vi "RemoveScanFunc.vi"(0 "LoadedInstIn":refnum<class "BaseDevice.lvclass">[](array[class]), 1 "LoadedFuncArr":string[](array[string]), 2 "ScanFunc":string, 3 "Multi ScanPar":bool[](array[boolean]), 5 "ScanSubPan":refnum<vi>, 7 "WholeTask(No:T)":bool, 9 "ScanFuncArrIn":string[][](array[string]), 11 "ErrorIn(No Error)":errorcluster caption="entrée d'erreur (pas d'erreur)", 12 "ActScanPar":bool[](array[boolean]), 13 "TaskIdx":i32) -> (4 "LoadedInst":refnum<class "BaseDevice.lvclass">[](array[class]), 6 "Multi ScanParOut":bool[](array[boolean]), 10 "ScanFuncArrOut":string[][](array[string]), 14 "ActScanParOut":bool[](array[boolean]), 15 "sortie d'erreur":errorcluster)   [LabVIEW 2019]
uses:
  DevicesClass/BaseDevice/BaseDevice.lvclass
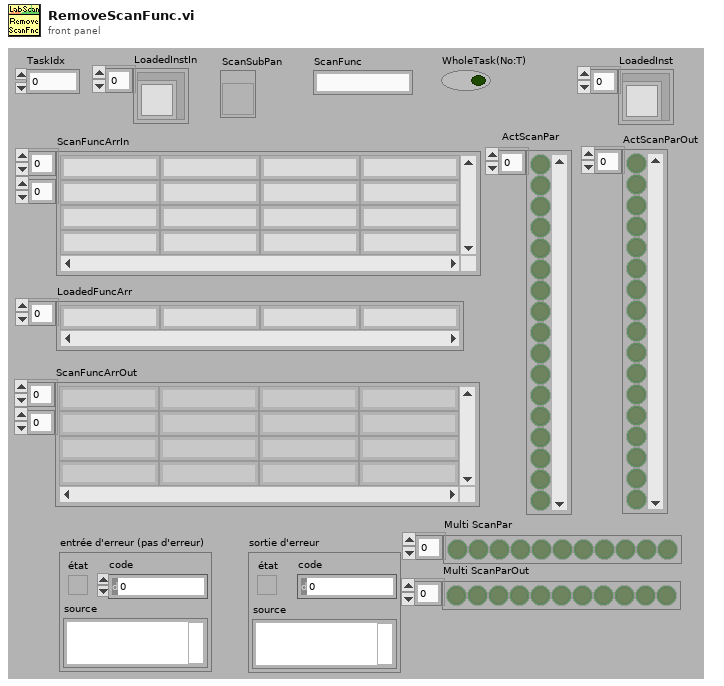
[diagram p1: front panel]
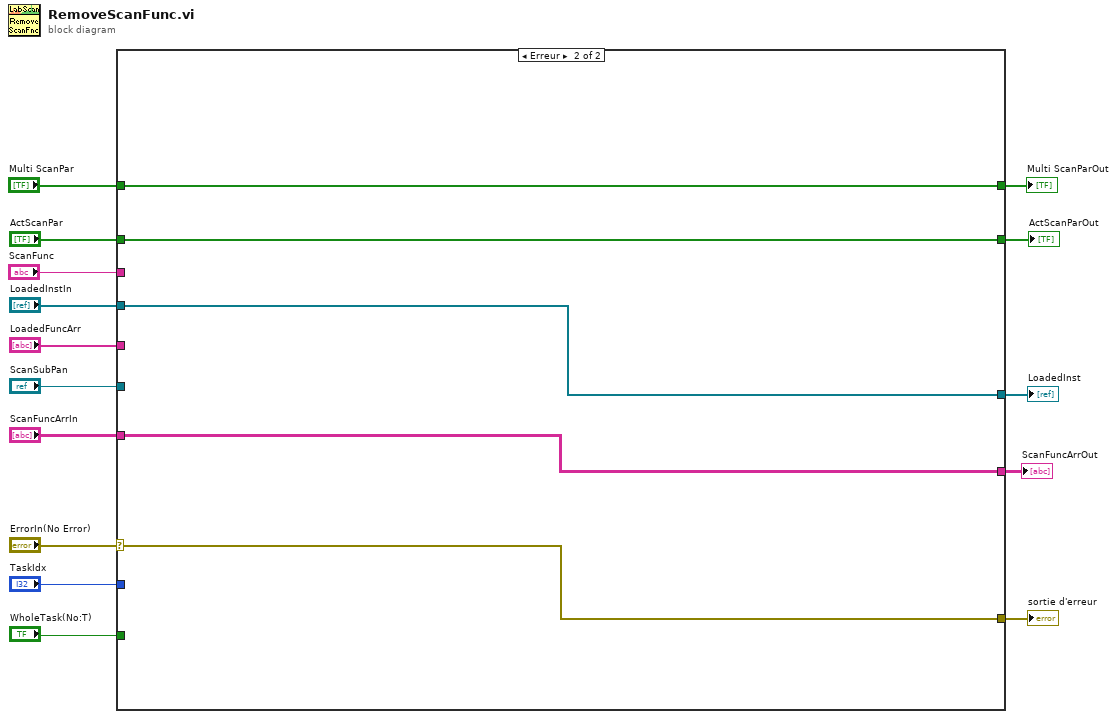
[diagram p0: block diagram]
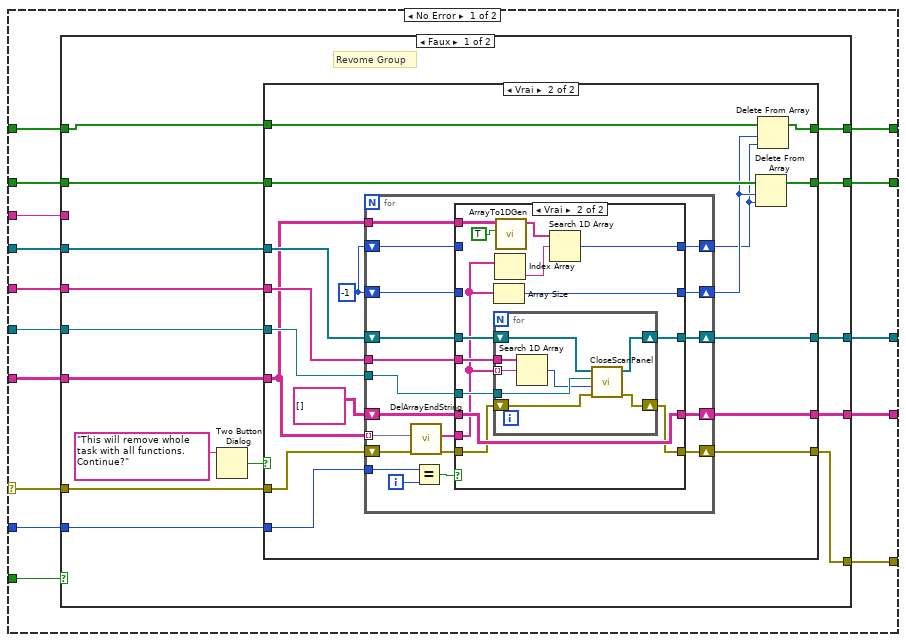
[diagram p2: hidden frame]
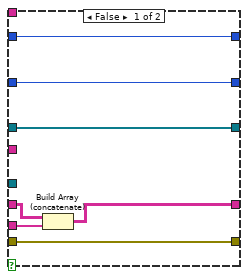
[diagram p4: hidden frame]
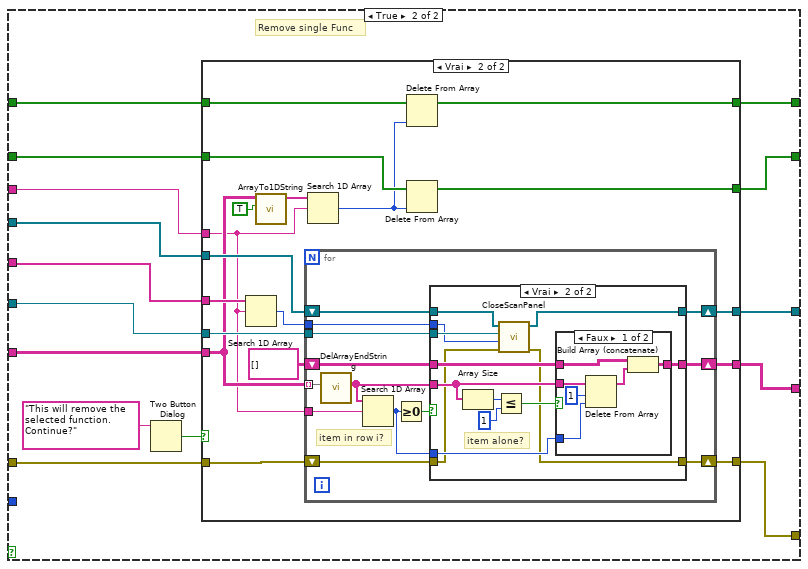
[diagram p5: hidden frame]
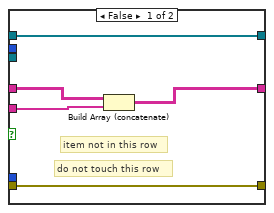
[diagram p7: hidden frame]
diagram:
  n1 = case shown="Erreur" "ErrorIn(No Error)" {
    selector: "ErrorIn(No Error)" -> [w30 w196]
    tunnel: "ScanFuncArrIn" -> [w27 w195]
    tunnel: "WholeTask(No:T)" -> [w28 _]
    tunnel: [w24 w196] -> w12
    tunnel: [w25 w195] -> w11
    tunnel: "ActScanPar" -> [w21 w194]
    tunnel: [w18 w194] -> w9
    tunnel: "TaskIdx" -> [w29 _]
    tunnel: [w26 w193] -> w7
    tunnel: "LoadedInstIn" -> [w23 w193]
    tunnel: "LoadedFuncArr" -> [w22 _]
    tunnel: "ScanSubPan" -> [w20 _]
    tunnel: "ScanFunc" -> [w19 _]
    tunnel: "Multi ScanPar" -> [w17 w192]
    tunnel: [w16 w192] -> w1
    frame No Error {
      n2 = case shown="Faux" w28 {
        tunnel: w27 -> [w42 w127]
        tunnel: w29 -> [w41 _]
        tunnel: w21 -> [w34 w121]
        tunnel: w30 -> [w44 w123]
        tunnel: [w40 w130] -> w26
        tunnel: [w39 w129] -> w25
        tunnel: [w38 w128] -> w24
        tunnel: w23 -> [w36 w125]
        tunnel: w22 -> [w37 w124]
        tunnel: w20 -> [w35 w126]
        tunnel: w19 -> [_ w122]
        tunnel: [w33 w120] -> w18
        tunnel: w17 -> [w32 w117]
        tunnel: [w31 w116] -> w16
        frame False {
          # "Revome Group"
          n3 = Two Button Dialog(message="This will remove whole task with all functions. Continue?") -> (T button?=w43:bool)  [unwired: 2 in]
          n4 = case shown="Vrai" w43 {
            tunnel: w42 -> [w50 w56]
            tunnel: w41 -> [_ w60]
            tunnel: [w50 w66] -> w39
            tunnel: w44 -> [w49 w67]
            tunnel: [w49 w65] -> w38
            tunnel: w36 -> [w48 w61]
            tunnel: w35 -> [_ w64]
            tunnel: w37 -> [_ w63]
            tunnel: [w48 w62] -> w40
            tunnel: w34 -> [w47 w59]
            tunnel: [w47 w58] -> w33
            tunnel: w32 -> [w46 w52]
            tunnel: [w46 w51] -> w31
            frame False {
              # "canceled"
            }
            frame True {
              w55 = -1
              n5 = for {
                tunnel: w56 -> [w83] mode=indexing
                shift-right: [w79] -> w66
                shift-left: string[][] [] -> [w80]
                tunnel: w60 -> [w84]
                shift-right: [w78] -> w65
                shift-left: w67 -> [w86]
                tunnel: w64 -> [w76]
                tunnel: w63 -> [w75]
                shift-right: [w74] -> w62
                shift-left: w61 -> [w73]
                shift-right: [w72] -> w54
                shift-left: w55 -> [w71]
                tunnel: w56 -> [w70]
                shift-right: [w69] -> w53
                shift-left: w55 -> [w68]
                i -> [w85]
                n6 = call <userlib>:"DelArrayEndString.vi"("ErrorIn(No Error)"=w86, "Array In"=w83) -> ("sortie d'erreur"=w77:errorcluster, "Array Out"=w81:string[])  [unwired: 8 in]
                n7 = Equal?(x=w84, y=w85) -> (x = y?=w82:bool)
                n8 = case shown="Vrai" w82 {
                  tunnel: w81 -> [w93 w99]
                  tunnel: w80 -> [w92 w106]
                  tunnel: [w91 w106] -> w79
                  tunnel: [w90 w102] -> w78
                  tunnel: w77 -> [w90 w103]
                  tunnel: w73 -> [w89 w104]
                  tunnel: w76 -> [_ w105]
                  tunnel: w75 -> [_ w107]
                  tunnel: [w89 w101] -> w74
                  tunnel: [w88 w100] -> w72
                  tunnel: w71 -> [w88 _]
                  tunnel: w70 -> [_ w98]
                  tunnel: [w87 w94] -> w69
                  tunnel: w68 -> [w87 _]
                  frame False {
                    n9 = Build Array (concatenate)(w92, w93) -> (w91:string[][])
                  }
                  frame True {
                    n10 = Array Size(array=w99) -> (size(s)=w100:i32)
                    n11 = for {
                      tunnel: w107 -> [w108]
                      tunnel: w99 -> [w115] mode=indexing
                      tunnel: w105 -> [w112]
                      shift-right: [w113] -> w102
                      shift-left: w103 -> [w114]
                      shift-right: [w109] -> w101
                      shift-left: w104 -> [w110]
                      n12 = Search 1D Array(1D array=w108, element=w115) -> (index of element=w111:i32)  [unwired: 1 in]
                      n13 = call "CloseScanPanel.vi"("error in (no error)"=w114, "Index"=w111, "SubPanRef"=w112, "LoadedInst"=w110) -> ("sortie d'erreur"=w113:errorcluster, "LoadedInst Out"=w109:refnum<class "BaseDevice.lvclass">[])  [unwired: 6 in]
                    }
                    n14 = Index Array(array=w99) -> (element=w95:string)  [unwired: 1 in]
                    n15 = call-poly <userlib>:"ArrayTo1DGen.vi"("DelArrEnd(F)"=TRUE, "tableau"=w98) -> ("Array Out"=w96:string[])  [unwired: 7 in, 2 out]
                    n16 = Search 1D Array(1D array=w96, element=w95) -> (index of element=w94:i32)  [unwired: 1 in]
                  }
                }
              }
              n17 = Delete From Array(array=w59, length=w54, index=w53) -> (array with subset deleted=w58:bool[])  [unwired: 1 out]
              n18 = Delete From Array(array=w52, length=w54, index=w53) -> (array with subset deleted=w51:bool[])  [unwired: 1 out]
            }
          }
        }
        frame True {
          # "Remove single Func"
          n19 = Two Button Dialog(message="This will remove the selected function. Continue?") -> (T button?=w118:bool)  [unwired: 2 in]
          n20 = case shown="Vrai" w118 {
            tunnel: w127 -> [w132 w145]
            tunnel: [w132 w152] -> w129
            tunnel: w122 -> [_ w143]
            tunnel: w125 -> [w135 w151]
            tunnel: w126 -> [_ w150]
            tunnel: w124 -> [_ w149]
            tunnel: [w133 w147] -> w128
            tunnel: [w135 w146] -> w130
            tunnel: w123 -> [w133 w142]
            tunnel: w121 -> [w134 w141]
            tunnel: [w134 w140] -> w120
            tunnel: w117 -> [w131 w138]
            tunnel: [w131 w136] -> w116
            frame False {
              # "canceled"
            }
            frame True {
              n21 = Search 1D Array(1D array=w149, element=w143) -> (index of element=w148:i32)  [unwired: 1 in]
              n22 = call <userlib>:"ArrayTo1DString.vi"("DelArrEnd(F)"=TRUE, "tableau"=w145) -> ("Array Out"=w144:string[])  [unwired: 7 in, 2 out]
              n23 = for {
                tunnel: w145 -> [w164] mode=indexing
                tunnel: w143 -> [w166]
                shift-right: [w161] -> w152
                shift-left: string[][] [] -> [w162]
                tunnel: w150 -> [w159]
                tunnel: w148 -> [w157]
                shift-right: [w155] -> w147
                shift-left: w142 -> [w156]
                shift-right: [w154] -> w146
                shift-left: w151 -> [w160]
                # "item in row i?"
                n24 = call <userlib>:"DelArrayEndString.vi"("Array In"=w164) -> ("Array Out"=w163:string[])  [unwired: 9 in, 1 out]
                n25 = Search 1D Array(1D array=w163, element=w166) -> (index of element=w158:i32)  [unwired: 1 in]
                n26 = Greater Or Equal To 0?(x=w158) -> (x >= 0?=w165:bool)
                n27 = case shown="Vrai" w165 {
                  tunnel: [w170 w180] -> w161
                  tunnel: w163 -> [w171 w179]
                  tunnel: w162 -> [w169 w181]
                  tunnel: w160 -> [w167 w174]
                  tunnel: w159 -> [_ w177]
                  tunnel: w158 -> [_ w178]
                  tunnel: w157 -> [_ w173]
                  tunnel: w156 -> [w168 w176]
                  tunnel: [w168 w175] -> w155
                  tunnel: [w167 w172] -> w154
                  frame False {
                    # "item not in this row"
                    # "do not touch this row"
                    n28 = Build Array (concatenate)(w169, w171) -> (w170:string[][])
                  }
                  frame True {
                    # "item alone?"
                    n29 = Array Size(array=w179) -> (size(s)=w184:i32)
                    n30 = Less Or Equal?(x=w184, y=1) -> (x <= y?=w182:bool)
                    n31 = call "CloseScanPanel.vi"("error in (no error)"=w176, "Index"=w173, "SubPanRef"=w177, "LoadedInst"=w174) -> ("sortie d'erreur"=w175:errorcluster, "LoadedInst Out"=w172:refnum<class "BaseDevice.lvclass">[])  [unwired: 6 in]
                    n32 = case shown="Faux" w182 {
                      tunnel: w181 -> [w188 w191]
                      tunnel: [w186 w191] -> w180
                      tunnel: w179 -> [w189 _]
                      tunnel: w178 -> [w185 _]
                      frame False {
                        n33 = Delete From Array(array=w189, length=1 ("longueur"), index=w185) -> (array with subset deleted=w187:string[])  [unwired: 1 out]
                        n34 = Build Array (concatenate)(w188, w187) -> (w186:string[][])
                      }
                      frame True {
                        # "item not alone \ndelete row"
                      }
                    }
                  }
                }
              }
              n35 = Search 1D Array(1D array=w144, element=w143) -> (index of element=w137:i32)  [unwired: 1 in]
              n36 = Delete From Array(array=w138, index=w137) -> (array with subset deleted=w136:bool[])  [unwired: 1 in, 1 out]
              n37 = Delete From Array(array=w141, index=w137) -> (array with subset deleted=w140:bool[])  [unwired: 1 in, 1 out]
            }
          }
        }
      }
    }
    frame Error {
    }
  }
  "sortie d'erreur" <- w12
  "ScanFuncArrOut" <- w11
  "ActScanParOut" <- w9
  "LoadedInst" <- w7
  "Multi ScanParOut" <- w1
